vi "circular_shooter_angle_calc_v2.vi"(0 "Driver Input":dbl, 1 "Low Angle":bool, 2 "High Angle":bool, 3 "Stabalize Angle":bool, 4 "Save Angle":bool, 5 "Current Angle":dbl, 7 "Saved Angle Preset":bool) -> (14 "Motor Voltage Out":dbl, 19 "Saved Angle":dbl)   [LabVIEW 2012]
panel:
  in  "High Angle Value":dbl=17.5
  in  "Low Angle Value":dbl=6.5
  in  "D":dbl
  in  "I":dbl
  in  "P":dbl=100.0
  in  "Lower Bound":dbl
  in  "Upper Bound":dbl=35.0
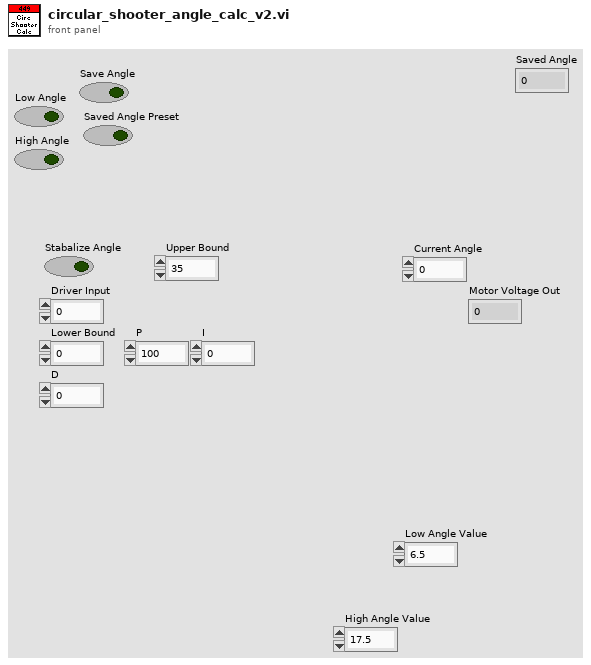
[diagram p1: front panel]
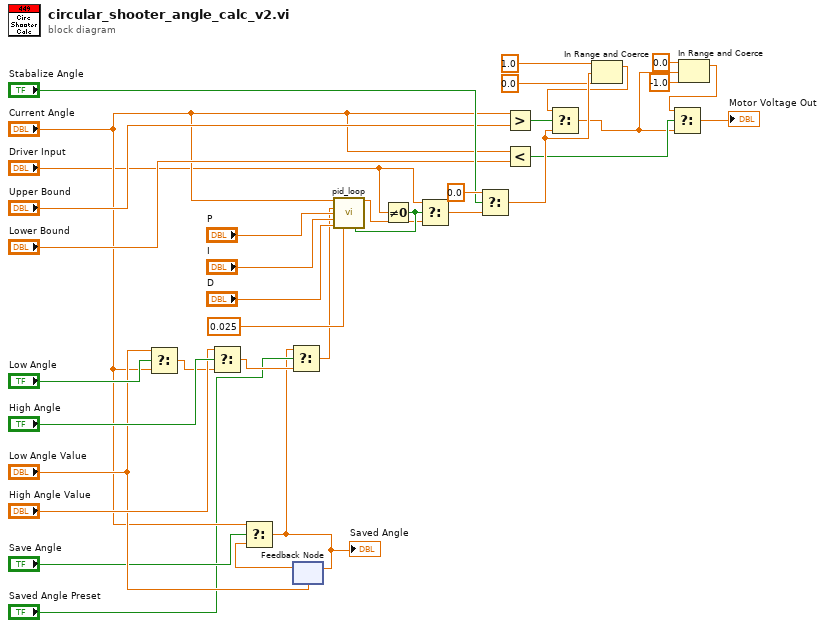
[diagram p0: block diagram]
diagram:
  n1 = Select(t="Low Angle Value", s="Low Angle", f="Current Angle") -> (s? t:f=w28:dbl)
  n2 = Select(t="High Angle Value", s="High Angle", f=w28) -> (s? t:f=w8:dbl)
  n3 = feedback #1("Low Angle Value") -> (w11:dbl)
  n4 = Select(t="Current Angle", s="Save Angle", f=w11) -> (s? t:f=w5:dbl)
  "Saved Angle" <- w5
  n5 = Select(t=w5, s="Saved Angle Preset", f=w8) -> (s? t:f=w7:dbl)
  n6 = feedback-in #1(w5) -> ()
  n7 = Not Equal To 0?(x="Driver Input") -> (x != 0?=w4:bool)
  n8 = call "pid_loop.vi"("Current Pos"="Current Angle", "Desired Pos"=w7, "P"="P", "I"="I", "D"="D", "dt"=0.025, "Reset ID"=w4) -> ("Voltage Output"=w2:dbl)  [unwired: 8 in]
  n9 = Select(t="Driver Input", s=w4, f=w2) -> (s? t:f=w1:dbl)
  n10 = Select(t=0.0, s="Stabalize Angle", f=w1) -> (s? t:f=w24:dbl)
  n11 = Greater?(x="Current Angle", y="Upper Bound") -> (0:w25:bool)
  n12 = Less?(x="Current Angle", y="Lower Bound") -> (x < y?=w17:bool)
  n13 = In Range and Coerce(upper limit=1.0, x=w24, lower limit=0.0) -> (coerced(x)=w23:dbl)  [unwired: 1 out]
  n14 = Select(t=w23, s=w25, f=w24) -> (s? t:f=w15:dbl)
  n15 = In Range and Coerce(upper limit=0.0, x=w15, lower limit=-1.0) -> (coerced(x)=w16:dbl)  [unwired: 1 out]
  n16 = Select(t=w16, s=w17, f=w15) -> (s? t:f=→"Motor Voltage Out":dbl)
